vi "mfd_status_text.vi"(8 "Refresh Rate (Hz)":u32=3) -> ()   [LabVIEW 2023]
uses:
  <vilib>/Utility/miscctls.llb/LVBoundsTypeDef.ctl
  mfd_global.vi
panel:
  out "MFD_StatusText":picture
  out "STATUSTEXT":T1(array[cluster])
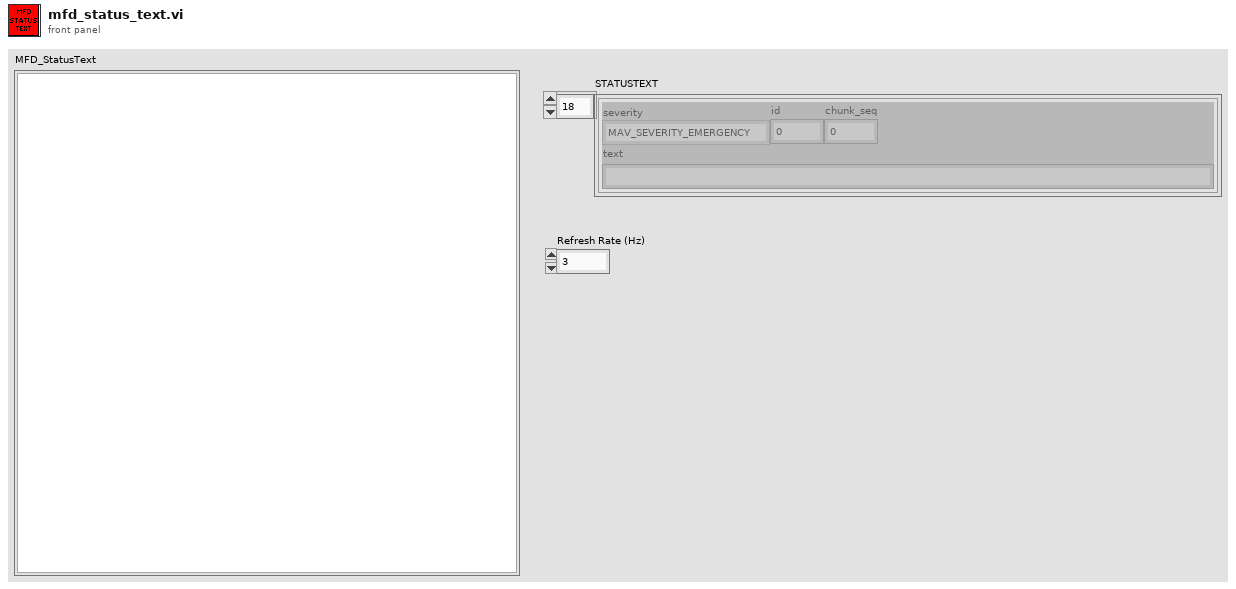
[diagram p1: front panel]
types:
  T1 = cluster{"severity":enum8{"MAV_SEVERITY_EMERGENCY", "MAV_SEVERITY_ALERT", "MAV_SEVERITY_CRITICAL", "MAV_SEVERITY_ERROR", "MAV_SEVERITY_WARNING", "MAV_SEVERITY_NOTICE", "MAV_SEVERITY_INFO", "MAV_SEVERITY_DEBUG"}, "id":u16, "chunk_seq":u8, "text":string}[]
  T2 = cluster{"Font Name:":string, "Size":i16, "Strikeout?":bool, "Italic?":bool, "Underline?":bool, "Outline?":bool, "Shadow?":bool, "Bold?":bool}
  T3 = enum16{"User-specified Font", "Application Font", "System Font", "Dialog Font"}
  T4 = cluster{"horizontal":enum16{"left", "center", "right"}, "vertical":enum16{"top", "center", "bottom"}}
  T5 = cluster{"left":i16, "top":i16, "right":i16, "bottom":i16}
  T6 = cluster{"Width":u16, "Style":enum32{"Solid", "Dash", "Dot", "DashDot", "DashDotDot"}}
  T7 = typedef "LVBoundsTypeDef.ctl" = cluster{"Width":u32, "Height":u32}
  T8 = typedef "imagedata.ctl" = cluster{"image type":i32, "image depth":i32, "image":u8[], "mask":u8[], "colors":u32[], "Rectangle":cluster{"left":i16, "top":i16, "right":i16, "bottom":i16}}
  T9 = cluster{"severity":bool, "id":bool, "chunk_seq":bool, "text":bool}[]
  T10 = enum8{"MAV_SEVERITY_EMERGENCY", "MAV_SEVERITY_ALERT", "MAV_SEVERITY_CRITICAL", "MAV_SEVERITY_ERROR", "MAV_SEVERITY_WARNING", "MAV_SEVERITY_NOTICE", "MAV_SEVERITY_INFO", "MAV_SEVERITY_DEBUG"}
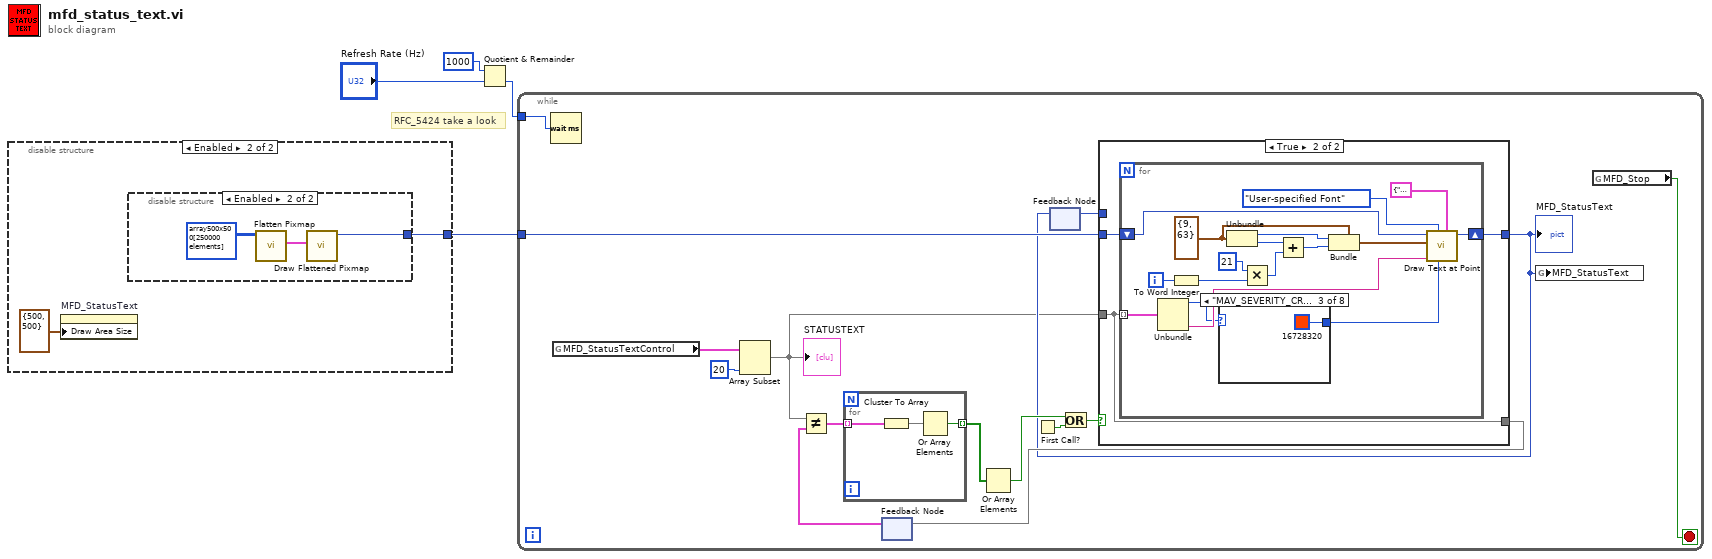
[diagram p0: block diagram]
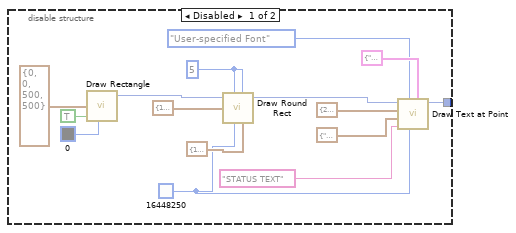
[diagram p2: hidden frame]
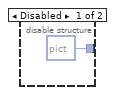
[diagram p3: hidden frame]
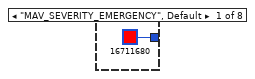
[diagram p5: hidden frame]
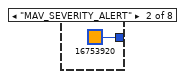
[diagram p6: hidden frame]
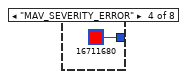
[diagram p7: hidden frame]
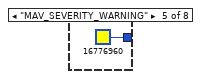
[diagram p8: hidden frame]
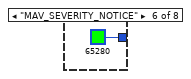
[diagram p9: hidden frame]
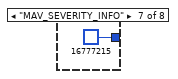
[diagram p10: hidden frame]
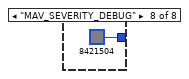
[diagram p11: hidden frame]
diagram:
  # "RFC_5424 take a look"
  n1 = disable-structure shown="Enabled" {
    disable-tunnel: [w5 w21] -> w4
    frame Disabled {
      w12 = u32 16448250 ("text color(black)")
      w15 = i16 5 ("oval height")
      n2 = call <vilib>:"Draw Rectangle.vi"("rect"=T5 {"left"=0, "top"=0, "right"=500, "bottom"=500}, "fill?(F)"=TRUE, "color(black)"=u32 0) -> ("new picture"=w16:picture)  [unwired: 6 in]
      n3 = call <vilib>:"Draw Round Rect.vi"("picture"=w16, "oval width"=w15, "rect"=T5 {"left"=172, "top"=17, "right"=329, "bottom"=47} ("rect 2"), "color(black)"=w12, "oval height"=w15, "pen"=T6 {"Width"=1, "Style"=enum."Solid"}) -> ("new picture"=w6:picture)  [unwired: 3 in]
      n4 = call <vilib>:"Draw Text at Point.vi"("[user-specified font]"=T2 {"Font Name:"="r", "Size"=25, "Strikeout?"=FALSE, "Italic?"=FALSE, "Underline?"=FALSE, "Outline?"=FALSE, "Shadow?"=FALSE, "Bold?"=TRUE}, "text color(black)"=w12, "desired font(Application)"=T3."User-specified Font", "text"="STATUS TEXT", "alignment(left, top)"=T4 {"horizontal"=enum."center", "vertical"=enum."top"}, "origin"=cluster{"x":i16, "y":i16} {"x"=250, "y"=20}, "picture"=w6) -> ("new picture"=w5:picture)  [unwired: 3 in, 1 out]
    }
    frame Enabled {
      n5 = property on="MFD_StatusText" class="Pict"("Draw Area Size"=T7 {"Width"=500, "Height"=500}) -> ()  [unwired: 2 in, 2 out]
      n6 = disable-structure shown="Enabled" {
        disable-tunnel: [picture bytes[150] ("new picture") w23] -> w21
        frame Disabled {
        }
        frame Enabled {
          n7 = call <vilib>:"Flatten Pixmap.vi"("24-bit pixmap"=u32[][] array500x500[250000 elements]) -> ("image data"=w24:T8)  [unwired: 10 in]
          n8 = call <vilib>:"Draw Flattened Pixmap.vi"("image data"=w24) -> ("new picture"=w23:picture)  [unwired: 8 in]
        }
      }
    }
  }
  n9 = Quotient & Remainder(x=u32 1000, y="Refresh Rate (Hz)") -> (floor(x/y)=w1:u32)  [unwired: 1 out]
  n10 = while {
    tunnel: w4 -> [w40]
    tunnel: w1 -> [w31]
    stop <- w30 stop-if-true
    n11 = Wait (ms)(milliseconds to wait=w31) -> ()  [unwired: 1 out]
    n12 = global read "mfd_global.vi" "MFD_StatusTextControl"() -> (w28:T1)
    n13 = Array Subset(array=w28, length=20) -> (w26:T1)  [unwired: 1 in]
    "STATUSTEXT" <- w26
    n14 = feedback #1() -> (w38:T1)  [unwired: 1 in]
    n15 = Not Equal?(x=w26, y=w38) -> (x != y?=w36:T9)
    n16 = for {
      tunnel: w36 -> [w43] mode=indexing
      tunnel: [w41] -> w35 mode=indexing
      n17 = Cluster To Array(cluster=w43) -> (array=w42:bool[])
      n18 = Or Array Elements(Boolean array=w42) -> (logical OR=w41:bool)
    }
    n19 = Or Array Elements(Boolean array=w35) -> (logical OR=w34:bool)
    n20 = First Call?() -> (First Call?: T/F=w32:bool)
    n21 = feedback #2() -> (w37:picture)  [unwired: 1 in]
    n22 = Or(x=w34, y=w32) -> (x .or. y?=w33:bool)
    n23 = case shown="True" w33 {
      tunnel: w40 -> [_ w48]
      tunnel: [w44 w47] -> w29
      tunnel: w26 -> [w45 w46]
      tunnel: [w45 w46] -> w39
      tunnel: w37 -> [w44 _]
      frame False {
      }
      frame True {
        n24 = for {
          tunnel: w46 -> [w49] mode=indexing
          shift-right: [w63] -> w47
          shift-left: w48 -> [w64]
          i -> [w54]
          w62 = cluster{"x":i16, "y":i16} {"x"=9, "y"=63} ("origin")
          n25 = Unbundle(w49) -> ("severity"=w51:T10, "text"=w52:string)  [unwired: 2 out]
          n26 = To Word Integer(number=w54) -> (16bit integer=w53:i16)
          n27 = case shown="\"MAV_SEVERITY_CRITICAL\"" w51 {
            tunnel: [u32 16711680 ("text color(black)") u32 16753920 ("text color(black)") u32 16728320 ("text color(black)") u32 16711680 ("text color(black)") u32 16776960 ("text color(black)") u32 65280 ("text color(black)") u32 16777215 ("text color(black)") u32 8421504 ("text color(black)")] -> w50
            frame "MAV_SEVERITY_EMERGENCY", Default {
            }
            frame "MAV_SEVERITY_ALERT" {
            }
            frame "MAV_SEVERITY_CRITICAL" {
            }
            frame "MAV_SEVERITY_ERROR" {
            }
            frame "MAV_SEVERITY_WARNING" {
            }
            frame "MAV_SEVERITY_NOTICE" {
            }
            frame "MAV_SEVERITY_INFO" {
            }
            frame "MAV_SEVERITY_DEBUG" {
            }
          }
          n28 = Unbundle(w62) -> ("x"=w60:i16, "y"=w55:i16)
          n29 = Multiply(x=i16 21 ("x 2"), y=w53) -> (x*y=w58:i16)
          n30 = Add(x=w55, y=w58) -> (x+y=w59:i16)
          n31 = Bundle(cluster=w62, "x"=w60, "y"=w59) -> (w61:cluster{"x":i16, "y":i16})
          n32 = call <vilib>:"Draw Text at Point.vi"("[user-specified font]"=T2 {"Font Name:"="g", "Size"=20, "Strikeout?"=FALSE, "Italic?"=FALSE, "Underline?"=FALSE, "Outline?"=FALSE, "Shadow?"=FALSE, "Bold?"=TRUE} ("[user-specified font] 2"), "text color(black)"=w50, "desired font(Application)"=T3."User-specified Font", "text"=w52, "origin"=w61, "picture"=w64) -> ("new picture"=w63:picture)  [unwired: 4 in, 1 out]
        }
      }
    }
    "MFD_StatusText" <- w29
    n33 = feedback-in #1(w39) -> ()
    n34 = feedback-in #2(w29) -> ()
    n35 = global write "mfd_global.vi" "MFD_StatusText"(w29) -> ()
    n36 = global read "mfd_global.vi" "MFD_Stop"() -> (w30:bool)
  }
